vi "Example.vi"() -> ()   [LabVIEW 2020]
uses:
  Single Weather.ctl
  BME280.lvclass
panel:
  in  "stop":bool
  out "Single Weather":T1
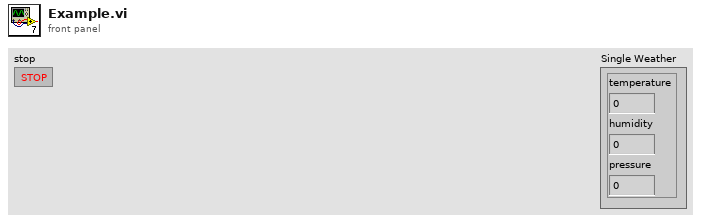
[diagram p1: front panel]
types:
  T1 = typedef "BME280.lvclass/Single Weather.ctl" = cluster{"temperature":dbl, "humidity":dbl, "pressure":dbl}
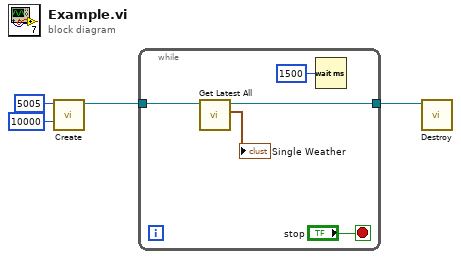
[diagram p0: block diagram]
diagram:
  n1 = call "Create.vi"("buffer"=10000, "port"=u16 5005) -> ("BME280 out"=w2:refnum<class "BME280.lvclass">)  [unwired: 8 in, 1 out]
  n2 = while {
    tunnel: w2 -> [w9]
    tunnel: [w8] -> w1
    stop <- "stop" stop-if-true
    n3 = call "Get Latest All.vi"("BME280 in"=w9) -> ("Single Weather"=→"Single Weather":T1, "BME280 out"=w8:refnum<class "BME280.lvclass">)  [unwired: 8 in, 1 out]
    n4 = Wait (ms)(milliseconds to wait=u32 1500) -> ()  [unwired: 1 out]
  }
  n5 = call "Destroy.vi"("BME280 in"=w1) -> ()  [unwired: 10 in, 1 out]
